vi "Delete Data (Stat Bundle).vi"(0 "Filepath":path, 1 "StartIndex":i32, 2 "EndIndex":i32, 3 "StatArray":string[][](array[string]), 5 "DataIndex":i32, 7 "StatIndex":i32, 11 "Error In":errorcluster) -> (15 "Error Out":errorcluster)   [LabVIEW 2013]
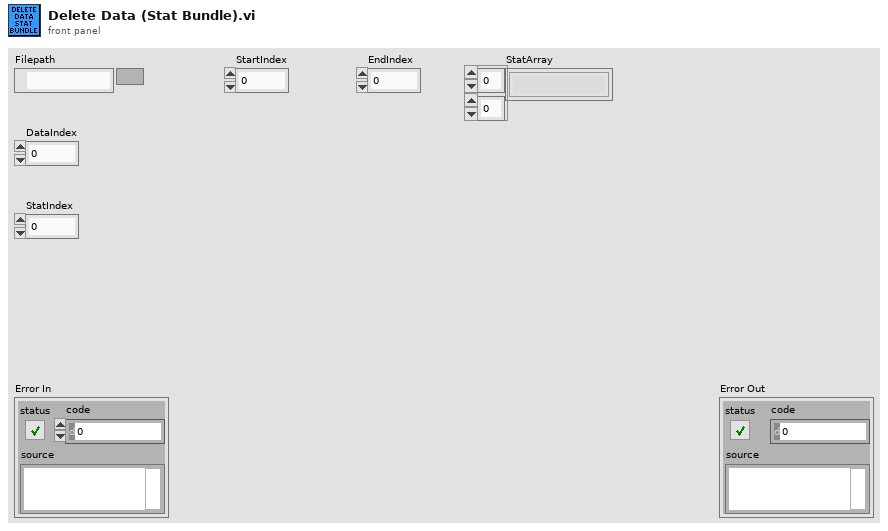
[diagram p1: front panel]
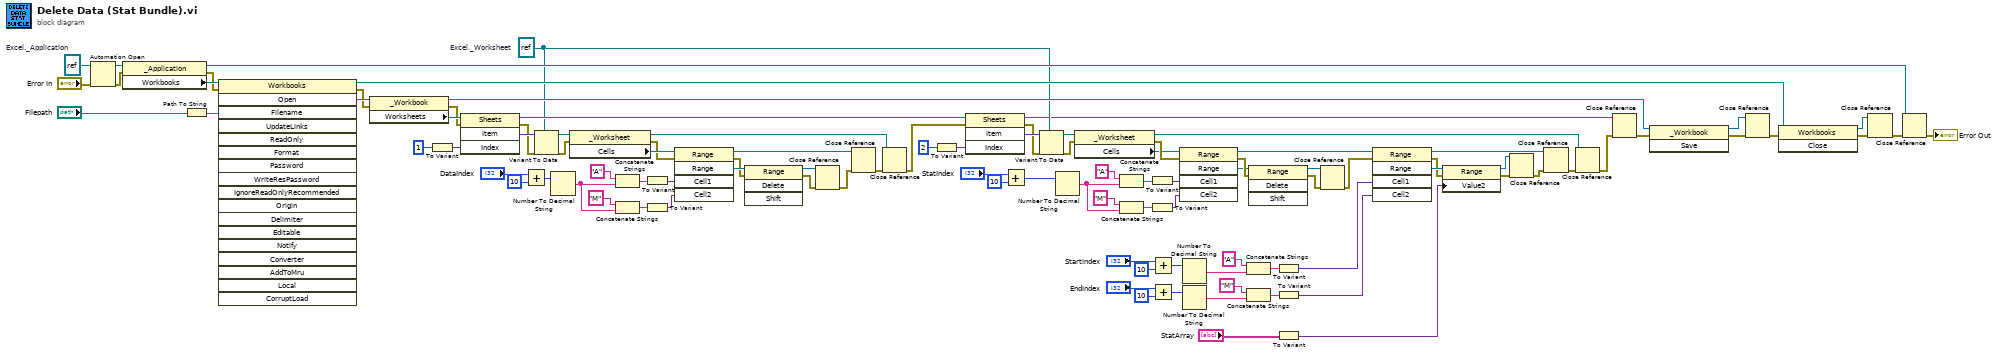
[diagram p0: block diagram]
diagram:
  w31 = refnum<k7> refnum  # Excel._Worksheet
  w99 = refnum<k7> refnum  # Excel._Application
  n1 = Automation Open(error in (no error)="Error In", Automation Refnum=w99) -> (Automation Refnum=w100:refnum<k7>, error out=w101:errorcluster)  [unwired: 2 in]
  n2 = property class="_Application"(reference=w100, error in=w101) -> (reference out=w92:refnum<k7>, error out=w93:errorcluster, "Workbooks"=w102:refnum<k7>)
  n3 = Path To String(path="Filepath") -> (string=w89:string)
  n4 = invoke class="Workbooks" method="Open"(reference=w102, error in=w93, "Filename"=w89) -> (reference out=w96:refnum<k7>, error out=w91:errorcluster, "Open"=w98:refnum<k7>)  [unwired: 15 in, 15 out]
  n5 = property class="_Workbook"(reference=w98, error in=w91) -> (reference out=w85:refnum<k7>, error out=w72:errorcluster, "Worksheets"=w73:refnum<k7>)
  n6 = To Variant(anything=1) -> (Variant=w81:variant)
  n7 = invoke class="Sheets" method="Item"(reference=w73, error in=w72, "Index"=w81) -> (reference out=w32:refnum<k7>, error out=w79:errorcluster, "Item"=w80:variant)  [unwired: 1 in, 1 out]
  n8 = Add(x="DataIndex", y=10) -> (x+y=w63:i32)
  n9 = Variant To Data(error in=w79, type=w31, Variant=w80) -> (data=w69:refnum<k7>, error out=w68:errorcluster)
  n10 = Number To Decimal String(number=w63) -> (decimal integer string=w58:string)  [unwired: 1 in]
  n11 = property class="_Worksheet"(reference=w69, error in=w68) -> (reference out=w77:refnum<k7>, error out=w70:errorcluster, "Cells"=w71:refnum<k7>)
  n12 = Concatenate Strings("A" ("ColumnIndex"), w58) -> (w56:string)
  n13 = Concatenate Strings("M" ("ColumnIndex"), w58) -> (w57:string)
  n14 = To Variant(anything=w56) -> (Variant=w74:variant)
  n15 = To Variant(anything=w57) -> (Variant=w66:variant)
  n16 = invoke class="Range" method="Range"(reference=w71, error in=w70, "Cell1"=w74, "Cell2"=w66) -> (reference out=w76:refnum<k7>, error out=w62:errorcluster, "Range"=w67:refnum<k7>)  [unwired: 1 in, 2 out]
  n17 = invoke class="Range" method="Delete"(reference=w67, error in=w62) -> (reference out=w61:refnum<k7>, error out=w60:errorcluster)  [unwired: 2 in, 2 out]
  n18 = Close Reference(reference=w61, error in (no error)=w60) -> (error out=w59:errorcluster)
  n19 = Close Reference(reference=w76, error in (no error)=w59) -> (error out=w78:errorcluster)
  n20 = Close Reference(reference=w77, error in (no error)=w78) -> (error out=w30:errorcluster)
  n21 = To Variant(anything=2) -> (Variant=w33:variant)
  n22 = invoke class="Sheets" method="Item"(reference=w32, error in=w30, "Index"=w33) -> (reference out=w29:refnum<k7>, error out=w28:errorcluster, "Item"=w34:variant)  [unwired: 1 in, 1 out]
  n23 = Add(x="StatIndex", y=10) -> (x+y=w26:i32)
  n24 = Variant To Data(error in=w28, type=w31, Variant=w34) -> (data=w41:refnum<k7>, error out=w42:errorcluster)
  n25 = Number To Decimal String(number=w26) -> (decimal integer string=w25:string)  [unwired: 1 in]
  n26 = property class="_Worksheet"(reference=w41, error in=w42) -> (reference out=w36:refnum<k7>, error out=w40:errorcluster, "Cells"=w39:refnum<k7>)
  n27 = Concatenate Strings("A" ("ColumnIndex"), w25) -> (w51:string)
  n28 = Concatenate Strings("M" ("ColumnIndex"), w25) -> (w50:string)
  n29 = To Variant(anything=w51) -> (Variant=w38:variant)
  n30 = To Variant(anything=w50) -> (Variant=w44:variant)
  n31 = Add(x="StartIndex", y=10) -> (x+y=w2:i32)
  n32 = Add(x="EndIndex", y=10) -> (x+y=w1:i32)
  n33 = invoke class="Range" method="Range"(reference=w39, error in=w40, "Cell1"=w38, "Cell2"=w44) -> (reference out=w24:refnum<k7>, error out=w47:errorcluster, "Range"=w43:refnum<k7>)  [unwired: 1 in, 2 out]
  n34 = Number To Decimal String(number=w2) -> (decimal integer string=w22:string)  [unwired: 1 in]
  n35 = Number To Decimal String(number=w1) -> (decimal integer string=w17:string)  [unwired: 1 in]
  n36 = Concatenate Strings("A" ("ColumnIndex"), w22) -> (w20:string)
  n37 = Concatenate Strings("M" ("ColumnIndex"), w17) -> (w21:string)
  n38 = invoke class="Range" method="Delete"(reference=w43, error in=w47) -> (reference out=w48:refnum<k7>, error out=w49:errorcluster)  [unwired: 2 in, 2 out]
  n39 = To Variant(anything=w20) -> (Variant=w16:variant)
  n40 = To Variant(anything=w21) -> (Variant=w15:variant)
  n41 = To Variant(anything="StatArray") -> (Variant=w12:variant)
  n42 = Close Reference(reference=w48, error in (no error)=w49) -> (error out=w23:errorcluster)
  n43 = invoke class="Range" method="Range"(reference=w24, error in=w23, "Cell1"=w16, "Cell2"=w15) -> (reference out=w8:refnum<k7>, error out=w11:errorcluster, "Range"=w14:refnum<k7>)  [unwired: 1 in, 2 out]
  n44 = property class="Range"(reference=w14, error in=w11, "Value2"=w12) -> (reference out=w9:refnum<k7>, error out=w10:errorcluster)
  n45 = Close Reference(reference=w9, error in (no error)=w10) -> (error out=w7:errorcluster)
  n46 = Close Reference(reference=w8, error in (no error)=w7) -> (error out=w35:errorcluster)
  n47 = Close Reference(reference=w36, error in (no error)=w35) -> (error out=w27:errorcluster)
  n48 = Close Reference(reference=w29, error in (no error)=w27) -> (error out=w90:errorcluster)
  n49 = invoke class="_Workbook" method="Save"(reference=w85, error in=w90) -> (reference out=w86:refnum<k7>, error out=w87:errorcluster)  [unwired: 1 in, 1 out]
  n50 = Close Reference(reference=w86, error in (no error)=w87) -> (error out=w88:errorcluster)
  n51 = invoke class="Workbooks" method="Close"(reference=w96, error in=w88) -> (reference out=w95:refnum<k7>, error out=w94:errorcluster)  [unwired: 1 in, 1 out]
  n52 = Close Reference(reference=w95, error in (no error)=w94) -> (error out=w97:errorcluster)
  n53 = Close Reference(reference=w92, error in (no error)=w97) -> (error out=→"Error Out":errorcluster)
